vi "FestoCPX.DI.Data.Fglb.vi"(6 "Config":T1[](array[typedef]), 7 "state (get)":T3=enum."get", 8 "error in (no error)":errorcluster, 9 "data bool":bool[](array[boolean]), 10 "data bytes":u8[](array[numeric]) format="%.0x") -> (0 "error out":errorcluster, 1 "data OR":bool[](array[boolean]), 2 "data out":bool[](array[boolean]), 3 "FrameCounter":i32, 4 "data AND":bool[](array[boolean]))   [LabVIEW 2016]
uses:
  FestoCPX.DI.Data.Fglb.Action.ctl
  FestoCPX.DI.Sets.ctl
  FestoCPX.DI.ctl
panel:
  out "DataIdx":i32
  out "dbg":bool[][](array[boolean])
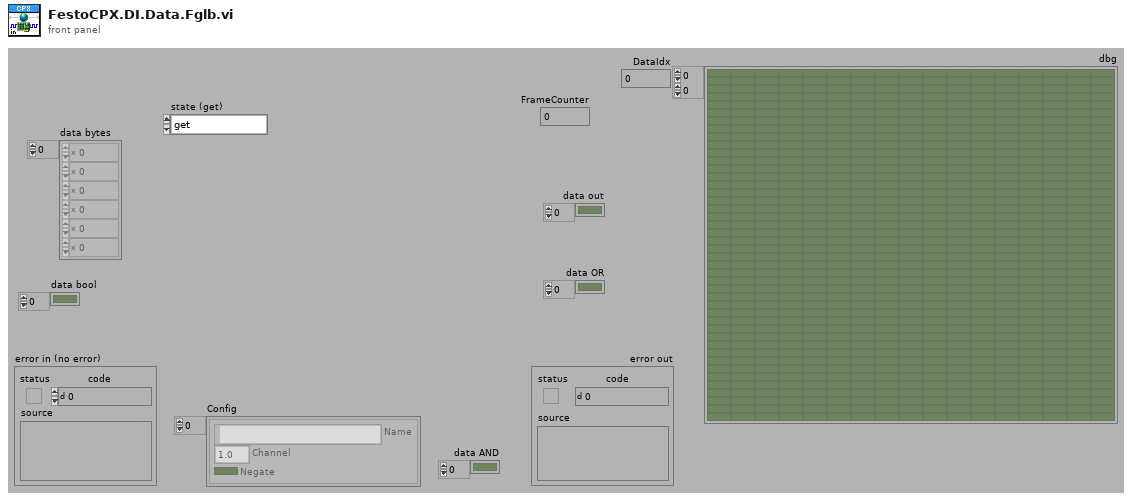
[diagram p1: front panel]
types:
  T1 = typedef "FestoCPX.DI.Sets.ctl" = cluster{"Name":string, "Channel":T2, "Negate":bool}
  T2 = typedef "FestoCPX.DI.ctl" = enum16{"0.0", "0.1", "0.2", "0.3", "0.4", "0.5", "0.6", "0.7", "1.0", "1.1", "1.2", "1.3", "1.4", "1.5", "1.6", "1.7", "2.0", "2.1", "2.2", "2.3", "2.4", "2.5", "2.6", "2.7", "3.0", "3.1", "3.2", "3.3", "3.4", "3.5", "3.6", "3.7", "4.0", "4.1", "4.2", "4.3", "4.4", "4.5", "4.6", "4.7"}
  T3 = typedef "FestoCPX.DI.Data.Fglb.Action.ctl" = enum16{"init", "set", "simul", "get"}
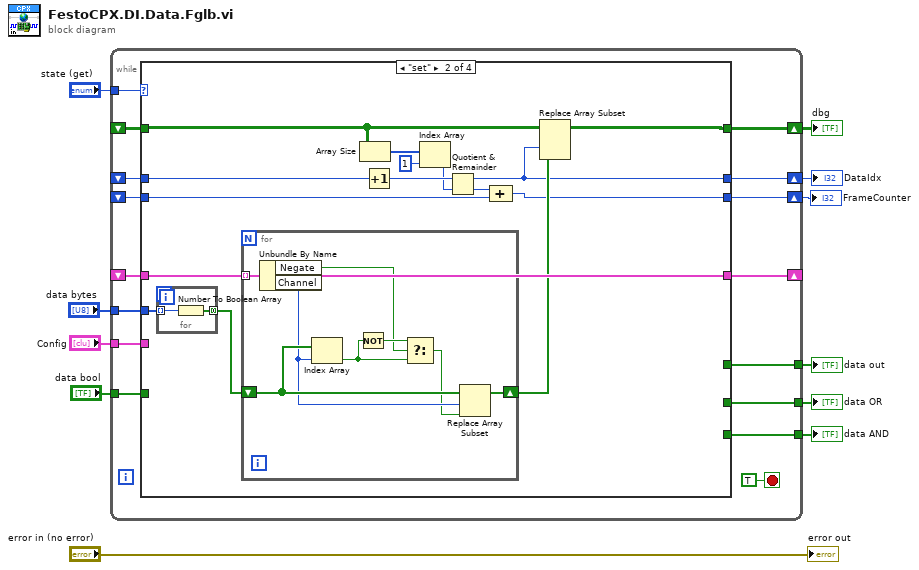
[diagram p0: block diagram]
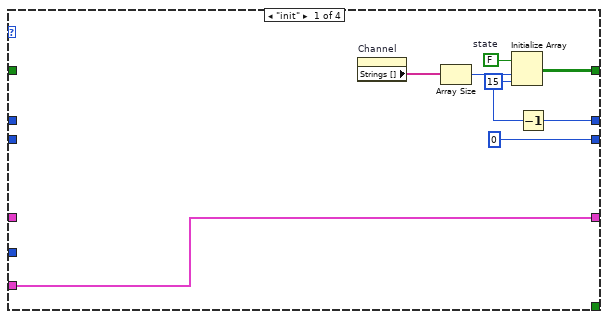
[diagram p2: hidden frame]
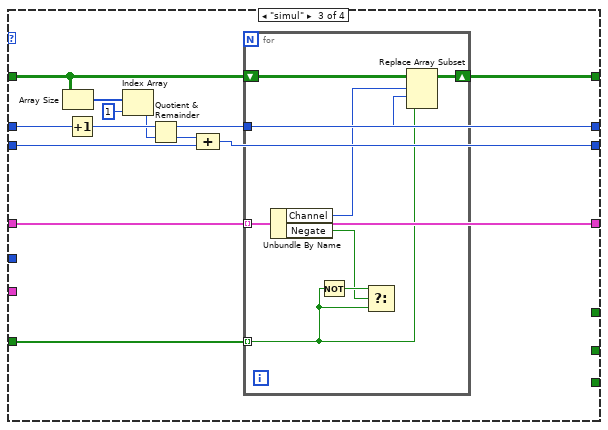
[diagram p3: hidden frame]
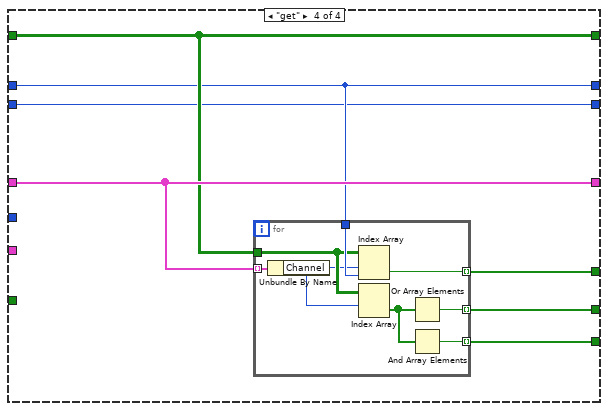
[diagram p4: hidden frame]
diagram:
  n1 = while {
    tunnel: "state (get)" -> [w26]
    shift-right: [w25] -> w3
    shift-left: _ -> [w24]
    tunnel: [w23] -> w8
    tunnel: "data bool" -> [w22]
    shift-right: [w21] -> _
    shift-left: _ -> [w20]
    tunnel: "Config" -> [w19]
    tunnel: "data bytes" -> [w18]
    shift-right: [w17] -> w2
    shift-left: _ -> [w16]
    tunnel: [w15] -> w5
    tunnel: [w14] -> w4
    shift-right: [w13] -> w1
    shift-left: _ -> [w12]
    stop <- TRUE stop-if-true
    n2 = case shown="\"set\"" w26 {
      tunnel: [w31 w41 w67 w87] -> w25
      tunnel: w24 -> [_ w40 w65 w87]
      tunnel: [_ _ _ w86] -> w23
      tunnel: w22 -> [_ _ w72 _]
      tunnel: [w35 w49 w73 w88] -> w21
      tunnel: w20 -> [_ w49 w73 w88]
      tunnel: w19 -> [w35 _ _ _]
      tunnel: w18 -> [_ w50 _ _]
      tunnel: [w29 w36 w66 w85] -> w17
      tunnel: w16 -> [_ w42 w64 w85]
      tunnel: [_ _ _ w84] -> w15
      tunnel: [_ _ _ w83] -> w14
      tunnel: [0 w37 w61 w82] -> w13
      tunnel: w12 -> [_ w38 w62 w82]
      frame "init" {
        w30 = 15 ("dimension size")
        w32 = FALSE  # state
        n3 = property on="Channel" class="Enum (strict)"() -> ("Strings []"=w34:string[])  [unwired: 2 in, 2 out]
        n4 = Array Size(array=w34) -> (size(s)=w33:i32)
        n5 = Initialize Array(w32, w33, w30) -> (w31:bool[][])
        n6 = Decrement(x=w30) -> (x-1=w29:i32)
      }
      frame "set" {
        n7 = for {
          tunnel: w50 -> [w60] mode=indexing
          tunnel: [w59] -> w48 mode=concatenating
          n8 = Number To Boolean Array(number=w60) -> (Boolean array=w59:bool[])
        }
        n9 = for {
          tunnel: w49 -> [w58] mode=indexing
          shift-right: [w51] -> w43
          shift-left: w48 -> [w54]
          n10 = Unbundle By Name(w58) -> ("Negate"=w56:bool, "Channel"=w53:T2)
          n11 = Index Array(array=w54, index=w53) -> (element=w55:bool)
          n12 = Not(x=w55) -> (.not. x?=w57:bool)
          n13 = Select(t=w57, s=w56, f=w55) -> (s? t:f=w52:bool)
          n14 = Replace Array Subset(array=w54, new element=w52, index=w53) -> (w51:bool[])
        }
        n15 = Array Size(array=w40) -> (size(s)=w47:i32[])
        n16 = Increment(x=w42) -> (x+1=w45:i32)
        n17 = Index Array(array=w47, index=1) -> (element=w44:i32)
        n18 = Quotient & Remainder(x=w45, y=w44) -> (x-y*floor(x/y)=w36:i32, floor(x/y)=w39:i32)
        n19 = Compound Arithmetic op=ADD(w39, w38) -> (w37:i32)
        n20 = Replace Array Subset(array=w40, new element=w43, index (col)=w36) -> (w41:bool[][])  [unwired: 1 in]
      }
      frame "simul" {
        n21 = Array Size(array=w65) -> (size(s)=w71:i32[])
        n22 = Increment(x=w64) -> (x+1=w69:i32)
        n23 = Index Array(array=w71, index=1) -> (element=w68:i32)
        n24 = Quotient & Remainder(x=w69, y=w68) -> (x-y*floor(x/y)=w66:i32, floor(x/y)=w63:i32)
        n25 = Compound Arithmetic op=ADD(w63, w62) -> (w61:i32)
        n26 = for {
          tunnel: w73 -> [w81] mode=indexing
          tunnel: w72 -> [w76] mode=indexing
          shift-right: [w78] -> w67
          shift-left: w65 -> [w77]
          tunnel: w66 -> [w75]
          n27 = Unbundle By Name(w81) -> ("Channel"=w74:T2, "Negate"=w79:bool)
          n28 = Not(x=w76) -> (.not. x?=w80:bool)
          n29 = Select(t=w80, s=w79, f=w76) -> ()  [unwired: 1 out]
          n30 = Replace Array Subset(array=w77, new element=w76, index (row)=w74, index (col)=w75) -> (w78:bool[][])
        }
      }
      frame "get" {
        n31 = for {
          tunnel: w87 -> [w93]
          tunnel: w88 -> [w96] mode=indexing
          tunnel: [w95] -> w86 mode=indexing
          tunnel: w85 -> [w94]
          tunnel: [w91] -> w84 mode=indexing
          tunnel: [w90] -> w83 mode=indexing
          n32 = Unbundle By Name(w96) -> ("Channel"=w92:T2)
          n33 = Index Array(array=w93, index (row)=w92, index (col)=w94) -> (element=w95:bool)
          n34 = Index Array(array=w93, index (row)=w92) -> (element=w89:bool[])  [unwired: 1 in]
          n35 = Or Array Elements(Boolean array=w89) -> (logical OR=w91:bool)
          n36 = And Array Elements(Boolean array=w89) -> (logical AND=w90:bool)
        }
      }
    }
  }
  "data out" <- w8
  "data OR" <- w5
  "data AND" <- w4
  "dbg" <- w3
  "DataIdx" <- w2
  "FrameCounter" <- w1
  "error out" <- "error in (no error)"
